vi "test1_korras.vi"() -> ()   [LabVIEW 2012]
panel:
  out "XY Graph":cluster{timestamp[], dbl[]}(graph)
  in  "Path":path
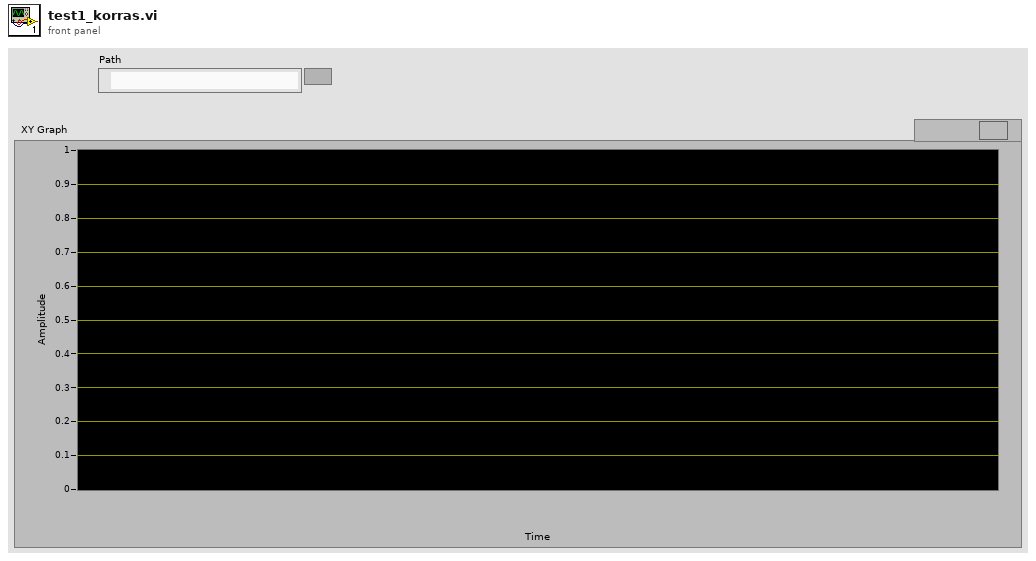
[diagram p1: front panel]
types:
  T1 = enum16{"open", "replace", "create", "open or create", "replace or create", "replace or create with confirmation"}
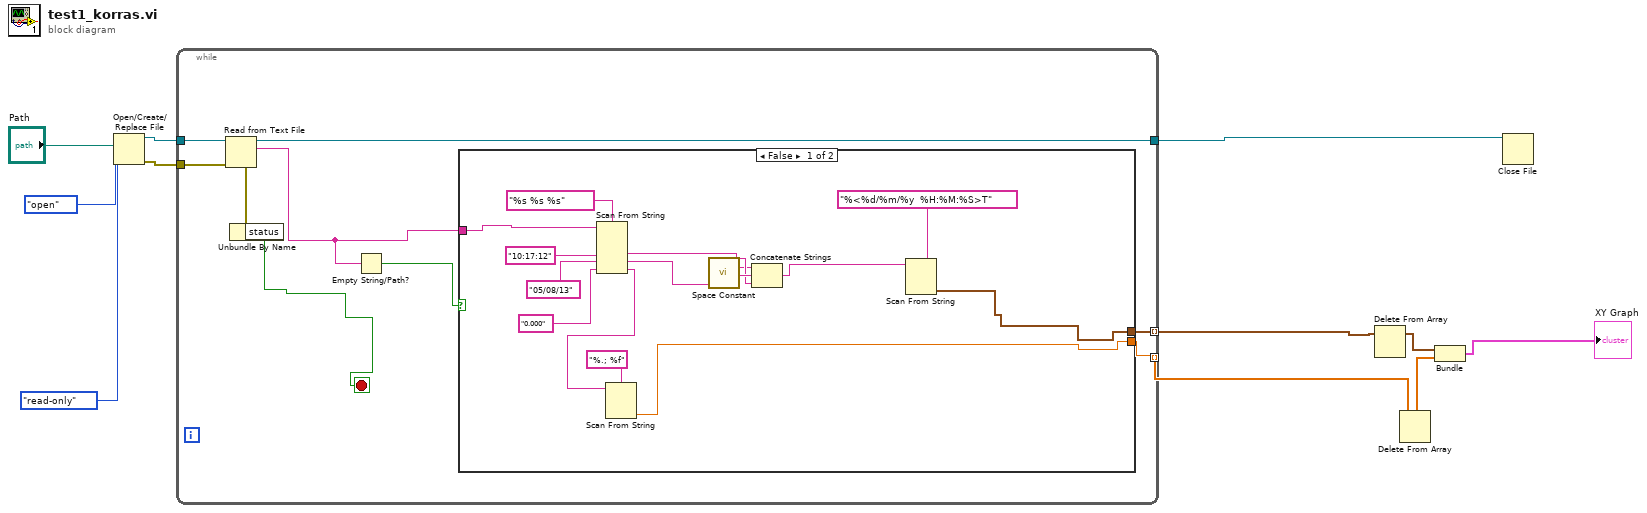
[diagram p0: block diagram]
diagram:
  n1 = Open/Create/Replace File(file path (use dialog)="Path", operation (0:open)=T1."open", access (0:read/write)=enum16{"read/write", "read-only", "write-only"}."read-only") -> (refnum out=w10:refnum<file>, error out=w11:errorcluster)  [unwired: 3 in, 1 out]
  n2 = while {
    tunnel: w11 -> [w20]
    tunnel: w10 -> [w18]
    tunnel: [w17] -> w6
    tunnel: [w15] -> w3 mode=indexing
    tunnel: [w16] -> w4 mode=indexing
    stop <- w12 stop-if-true
    n3 = Read from Text File(file (use dialog)=w18, error in=w20) -> (refnum out=w17:refnum<file>, text=w14:string, error out=w19:errorcluster)  [unwired: 2 in, 1 out]
    n4 = Unbundle By Name(w19) -> ("status"=w12:bool)
    n5 = Empty String/Path?(string/path=w14) -> (empty?=w13:bool)
    n6 = case shown="False" w13 {
      tunnel: [w22 _] -> w16
      tunnel: [w21 _] -> w15
      tunnel: w14 -> [w23 _]
      frame False {
        n7 = Scan From String(format string="%s %s %s", input string=w23, default 1="10:17:12", default 2="05/08/13", default 3="0.000") -> (output 1=w30:string, output 2=w29:string, output 3=w32:string)  [unwired: 2 in, 3 out]
        n8 = Scan From String(format string="%.; %f", input string=w32) -> (output 1=w21:dbl)  [unwired: 3 in, 3 out]
        n9 = call <vilib>:"Space Constant.vi"() -> ("String"=w31:string)
        n10 = Concatenate Strings(w29, w31, w30) -> (w27:string)
        n11 = Scan From String "Scan From String"(format string="%<%d/%m/%y  %H:%M:%S>T", input string=w27) -> (output 1=w22:timestamp)  [unwired: 3 in, 3 out]
      }
      frame True {
      }
    }
  }
  n12 = Delete From Array(array=w4) -> (array with subset deleted=w1:timestamp[])  [unwired: 2 in, 1 out]
  n13 = Delete From Array(array=w3) -> (array with subset deleted=w2:dbl[])  [unwired: 2 in, 1 out]
  n14 = Bundle(w1, w2) -> (→"XY Graph":cluster{timestamp[], dbl[]})  [unwired: 1 in]
  n15 = Close File(refnum=w6) -> ()  [unwired: 1 in, 2 out]
